vi "IlluminationPatterns.vi"() -> ()   [LabVIEW 2011]
panel:
  in  "Illumination Patterns":T1(radio)
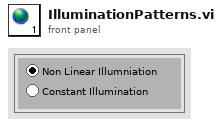
[diagram p1: front panel]
types:
  T1 = enum32{"Non Linear Illumniation", "Constant Illumination"}
diagram:
